vi "Enable VFD.vi"(6 "Direction":T1=2 items=["Reverse"=0, "Forward"=2], 8 "error In":errorcluster, 11 "Enable":bool) -> (0 "error out":errorcluster)   [LabVIEW 2026, in "VFD Library.lvlib"]
uses:
  VFD Library.lvlib
  Direction Selection.ctl
  Private/State Selection FGV.ctl
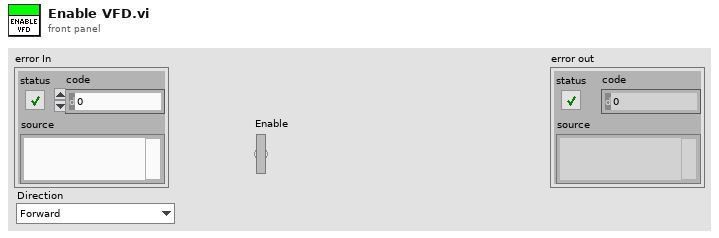
[diagram p1: front panel]
types:
  T1 = typedef "VFD Library.lvlib/Direction Selection.ctl" = u16
  T2 = typedef "State Selection FGV.ctl" = enum16{"Initilize", "Write Reg", "Write Multiple Reg", "Read Reg", "Write Coil", "Read Coil", "Reset", "Close"}
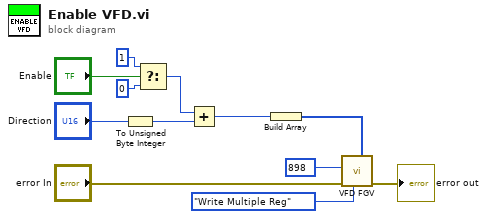
[diagram p0: block diagram]
diagram:
  n1 = To Unsigned Byte Integer(number="Direction") -> (unsigned 8bit integer=w3:u8)
  n2 = Select(t=u8 1 ("value"), s="Enable", f=u8 0 ("value")) -> (s? t:f=w5:u8)
  n3 = Add(x=w5, y=w3) -> (x+y=w2:u8)
  n4 = Build Array(w2) -> (w1:u8[])
  n5 = call "VFD FGV.vi"("values Mutiple Reg"=w1, "State"=State_Selection_FGV."Write Multiple Reg", "error In"="error In", "address"=u16 898) -> ("error out"=→"error out":errorcluster)  [unwired: 5 in, 2 out]
